vi "MemBlockTagList(LVObject).vi"(7 "方法":enum16{"初始化", "获取索引"}(ring), 8 "error in (no error)":errorcluster caption="错误输入（无错误）", 10 "标签":string, 11 "内存块标签列表":T1(array[cluster])) -> (0 "error out":errorcluster caption="错误输出", 1 "标签索引":i32, 3 "默认值":refnum<class>[](array[class]))   [LabVIEW 2013, in "MemBlock.lvlib"]
uses:
  MemBlock.lvlib
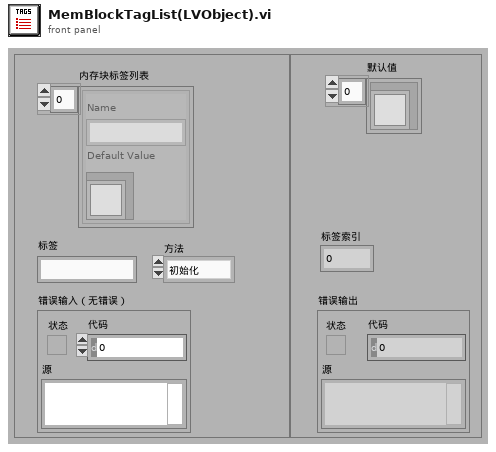
[diagram p1: front panel]
types:
  T1 = cluster{"Name":string, "Default Value":refnum<class>}[]
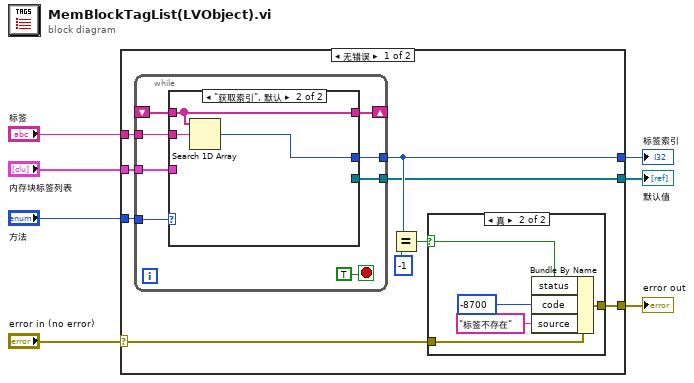
[diagram p0: block diagram]
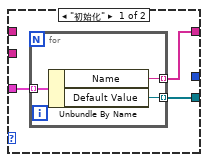
[diagram p3: hidden frame]
diagram:
  n1 = case shown="无错误" "error in (no error)" {
    selector: "error in (no error)" -> [w14 _]
    tunnel: [w13 _] -> w6
    tunnel: [w12 _] -> w5
    tunnel: [w11 _] -> w4
    tunnel: "内存块标签列表" -> [w10 _]
    tunnel: "标签" -> [w9 _]
    tunnel: "方法" -> [w8 _]
    frame No Error {
      n2 = while {
        shift-right: [w26] -> _
        shift-left: _ -> [w28]
        tunnel: w8 -> [w29]
        tunnel: w10 -> [w27]
        tunnel: [w25] -> w11
        tunnel: w9 -> [w24]
        tunnel: [w23] -> w12
        stop <- TRUE stop-if-true
        n3 = case shown="\"获取索引\", 默认" w29 {
          tunnel: w28 -> [_ w37]
          tunnel: w27 -> [w33 _]
          tunnel: [w32 w37] -> w26
          tunnel: [w31 _] -> w25
          tunnel: w24 -> [_ w39]
          tunnel: [_ w38] -> w23
          frame "初始化" {
            n4 = for {
              tunnel: w33 -> [w36] mode=indexing
              tunnel: [w35] -> w32 mode=indexing
              tunnel: [w34] -> w31 mode=indexing
              n5 = Unbundle By Name(w36) -> ("Name"=w35:string, "Default Value"=w34:refnum<class>)
            }
          }
          frame "获取索引", Default {
            n6 = Search 1D Array(1D array=w37, element=w39) -> (index of element=w38:i32)  [unwired: 1 in]
          }
        }
      }
      n7 = Equal?(x=w12, y=-1) -> (x = y?=w15:bool)
      n8 = case shown="真" w15 {
        selector: w15 -> [_ w22]
        tunnel: [w17 w21] -> w13
        tunnel: w14 -> [w17 w18]
        frame False {
        }
        frame True {
          n9 = Bundle By Name(cluster=w18, "status"=w22, "code"=-8700, "source"="标签不存在") -> (w21:errorcluster)
        }
      }
    }
    frame Error {
    }
  }
  "error out" <- w6
  "标签索引" <- w5
  "默认值" <- w4
